vi "CreateVIPictures.vi"(8 "error in (no error)":errorcluster, 9 "Capture Target":T3=enum."Front Panel", 10 "VI 1 Screenshots":T1, 11 "Picture Save Location":path) -> (0 "error out":errorcluster, 2 "Screenshot Files":path[](array[path]))   [LabVIEW 2015, in "VIDiffScreenshots.lvlib"]
doc: "Captures .png imgaes of the VI given the path and the picture configuration."
uses:
  VIDiffScreenshots.lvlib
  Screenshot Type.ctl
  VIScreenshots.ctl
  ScreenshotInfo.ctl
  Utilities/FilePaths.ctl
  Utilities/VIDiffUtilities.lvlib
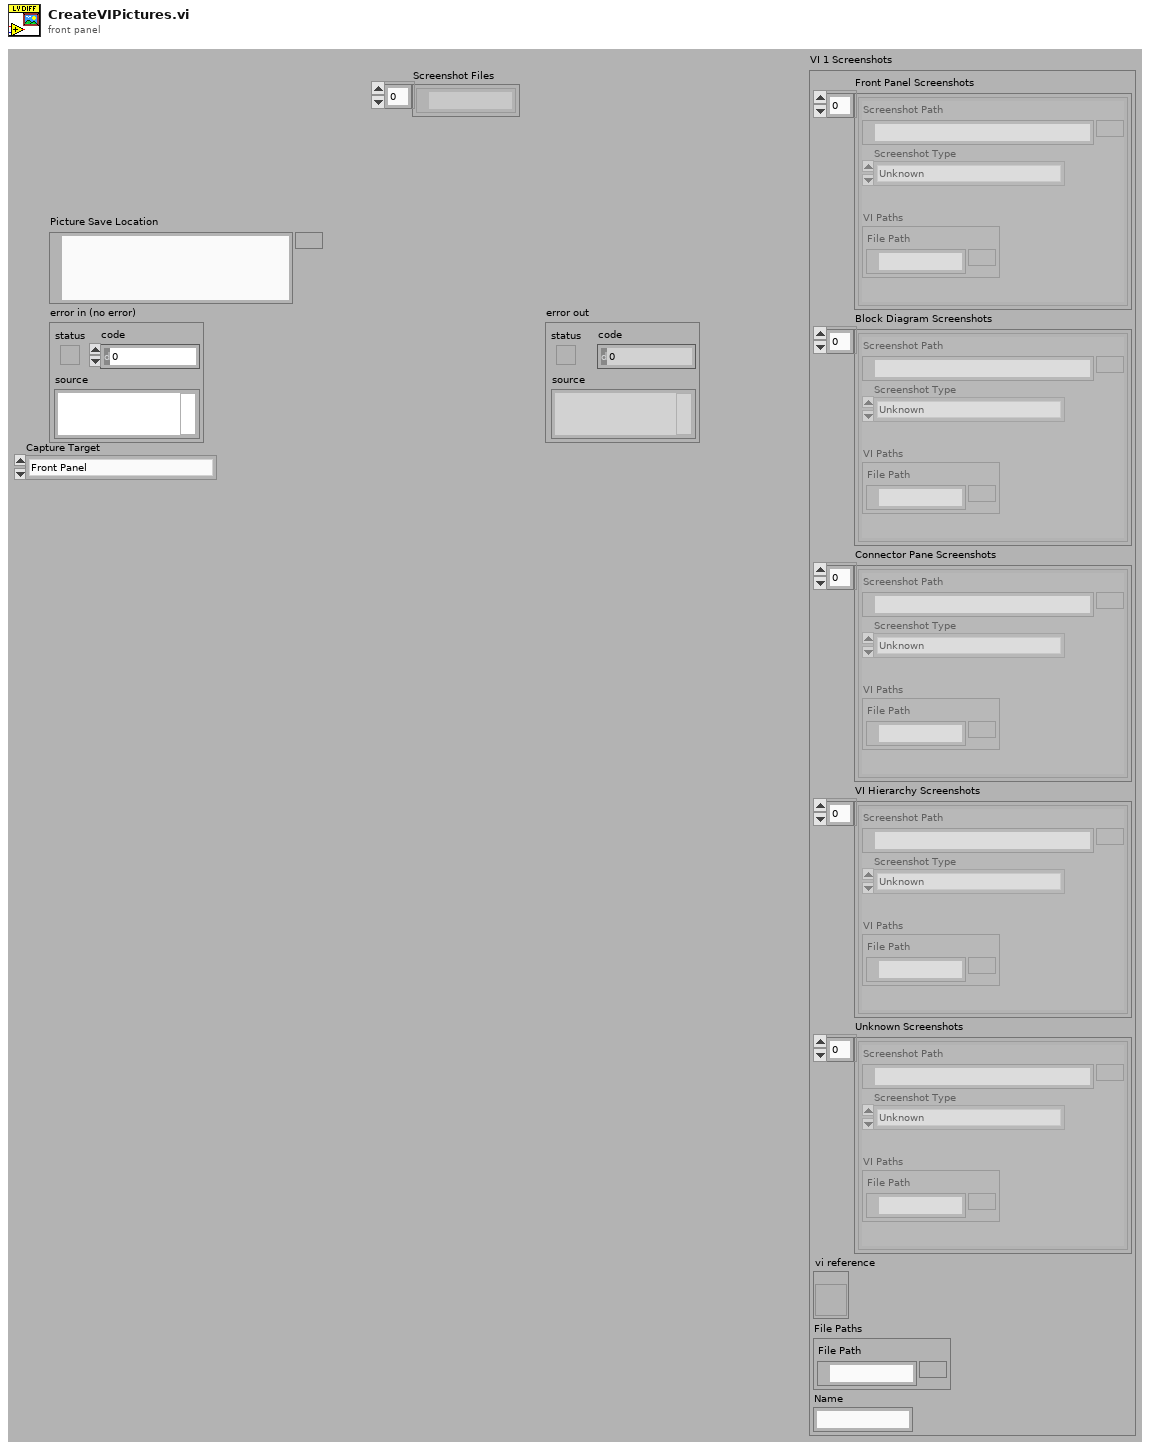
[diagram p1: front panel]
types:
  T1 = typedef "VIDiffScreenshots.lvlib/VIScreenshots.ctl" = cluster{"Front Panel Screenshots":T2[], "Block Diagram Screenshots":T2[], "Connector Pane Screenshots":T2[], "VI Hierarchy Screenshots":T2[], "Unknown Screenshots":T2[], "vi reference":refnum<vi>, "File Paths":cluster{"File Path":path}, "Name":string}
  T2 = typedef "VIDiffScreenshots.lvlib/ScreenshotInfo.ctl" = cluster{"Screenshot Path":path, "Screenshot Type":T3, "VI Paths":T4}
  T3 = typedef "VIDiffScreenshots.lvlib/Screenshot Type.ctl" = enum16{"Unknown", "Front Panel", "Connector Pane", "Block Diagram", "VI Hierarchy"}
  T4 = typedef "VIDiffUtilities.lvlib/FilePaths.ctl" = cluster{"File Path":path}
  T5 = cluster{"Printing:Custom All Controls?":bool, "Printing:Custom Connector?":bool, "Printing:Custom Control Descriptions?":bool, "Printing:Custom Control Types?":bool, "Printing:Custom Controls?":bool, "Printing:Custom Description?":bool, "Printing:Custom Diagram Hidden?":bool, "Printing:Custom Diagram Repeat?":bool, "Printing:Custom Diagram?":bool, "Printing:Custom Hierarchy?":bool, "Printing:Custom History?":bool, "Printing:Custom Panel Border?":bool, "Printing:Custom Panel?":bool, "Printing:Custom SubVIs?":bool}
  T6 = enum32{"Custom", "Standard", "Using Panel", "Using SubVI", "Complete"}
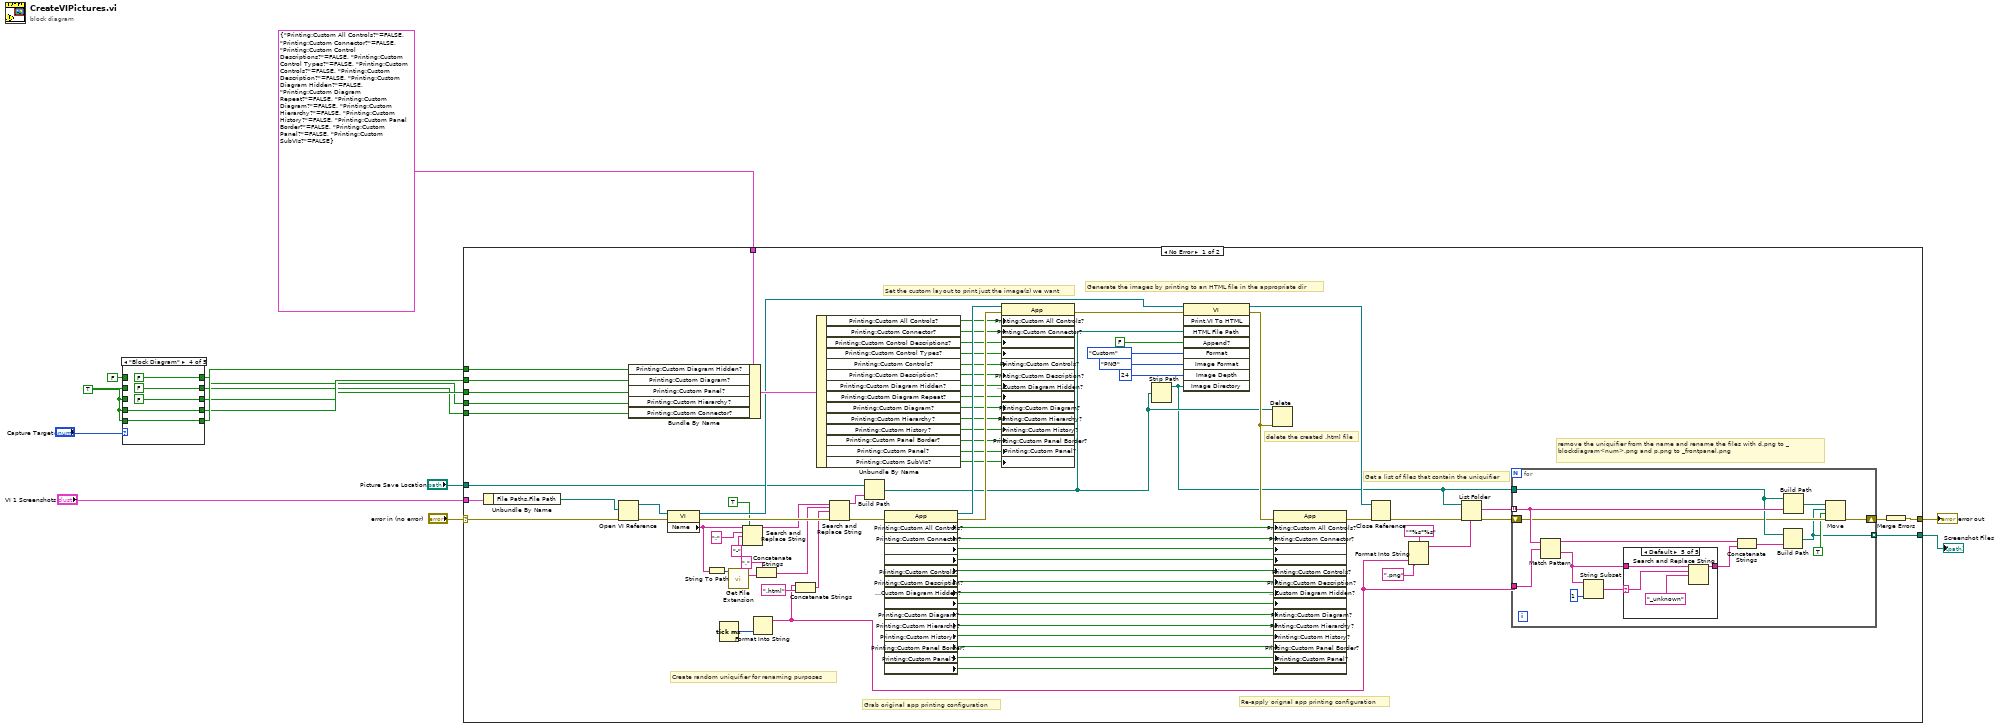
[diagram p0: block diagram]
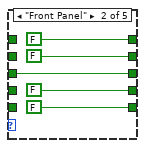
[diagram p3: hidden frame]
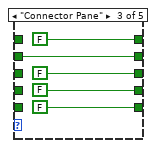
[diagram p4: hidden frame]
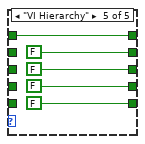
[diagram p5: hidden frame]
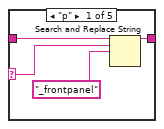
[diagram p6: hidden frame]
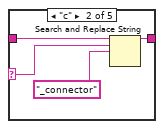
[diagram p7: hidden frame]
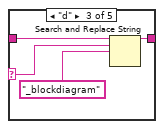
[diagram p8: hidden frame]
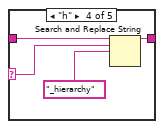
[diagram p9: hidden frame]
diagram:
  w6 = TRUE ("Capture Hierarchy?")
  n1 = case shown="\"Block Diagram\"" "Capture Target" {
    tunnel: FALSE ("Capture Hierarchy?") -> [w19 _ _ _ w35]
    tunnel: w6 -> [w18 _ w28 _ _]
    tunnel: w6 -> [w17 w24 _ _ _]
    tunnel: w6 -> [w16 _ _ w31 _]
    tunnel: w6 -> [w15 _ _ w30 _]
    tunnel: [w19 FALSE ("Capture Hierarchy?") FALSE ("Capture Hierarchy?") FALSE ("Capture Hierarchy?") w35] -> w2
    tunnel: [w18 FALSE ("Capture Connector?") w28 FALSE ("Capture Block Diagram?") FALSE ("Capture Block Diagram?")] -> w1
    tunnel: [w17 w24 FALSE ("Capture Block Diagram?") FALSE ("Capture Block Diagram?") FALSE ("Capture Block Diagram?")] -> w3
    tunnel: [w16 FALSE ("Capture Block Diagram?") FALSE ("Capture Block Diagram?") w31 FALSE ("Capture Block Diagram?")] -> w4
    tunnel: [w15 FALSE ("Capture Hidden Cases?") FALSE ("Capture Hidden Cases?") w30 FALSE ("Capture Block Diagram?")] -> w5
    frame "Unknown", Default {
    }
    frame "Front Panel" {
    }
    frame "Connector Pane" {
    }
    frame "Block Diagram" {
    }
    frame "VI Hierarchy" {
    }
  }
  n2 = case shown="No Error" "error in (no error)" {
    selector: "error in (no error)" -> [w43 w153]
    tunnel: T5 {"Printing:Custom All Controls?"=FALSE, "Printing:Custom Connector?"=FALSE, "Printing:Custom Control Descriptions?"=FALSE, "Printing:Custom Control Types?"=FALSE, "Printing:Custom Controls?"=FALSE, "Printing:Custom Description?"=FALSE, "Printing:Custom Diagram Hidden?"=FALSE, "Printing:Custom Diagram Repeat?"=FALSE, "Printing:Custom Diagram?"=FALSE, "Printing:Custom Hierarchy?"=FALSE, "Printing:Custom History?"=FALSE, "Printing:Custom Panel Border?"=FALSE, "Printing:Custom Panel?"=FALSE, "Printing:Custom SubVIs?"=FALSE} ("Content Options") -> [w118 _]
    tunnel: w5 -> [w117 _]
    tunnel: w4 -> [w116 _]
    tunnel: w3 -> [w115 _]
    tunnel: "Picture Save Location" -> [w74 _]
    tunnel: [w60 w153] -> w12
    tunnel: w2 -> [w59 _]
    tunnel: w1 -> [w58 _]
    tunnel: "VI 1 Screenshots" -> [w45 _]
    tunnel: [w41 _] -> w10
    frame No Error {
      # "remove the uniquifier from the name and rename the files with d.png to _blockdiagram<num>.png and p.png to _frontpanel.png"
      # "Get a list of files that contain the uniquifier"
      # "delete the created .html file"
      # "Create random uniquifier for renaming purposes"
      # "Re-apply orignal app printing configuration"
      # "Grab original app printing configuration"
      # "Generate the images by printing to an HTML file in the appropriate dir"
      # "Set the custom layout to print just the image(s) we want"
      n3 = Unbundle By Name(w45) -> ("File Paths.File Path"=w44:path)
      n4 = Open VI Reference(vi path=w44, error in (no error)=w43) -> (vi reference=w77:refnum<vi>, error out=w75:errorcluster)  [unwired: 4 in]
      n5 = Bundle By Name(cluster=w118, "Printing:Custom Diagram Hidden?"=w117, "Printing:Custom Diagram?"=w116, "Printing:Custom Panel?"=w115, "Printing:Custom Hierarchy?"=w59, "Printing:Custom Connector?"=w58) -> (w81:T5)
      n6 = property class="VI"(reference=w77, error in=w75) -> (reference out=w76:refnum<vi>, error out=w69:errorcluster, "Name"=w53:string)
      n7 = String To Path(string=w53) -> (path=w57:path)
      n8 = Tick Count (ms)() -> (millisecond timer value=w42:u32)
      n9 = call <vilib>:"Get File Extension.vi"("file"=w57) -> ("lowercase file extension"=w56:string)  [unwired: 6 in, 4 out]
      n10 = Search and Replace String(replace all?=TRUE ("replace all? (F)"), input string=w53, search string=":", replace string="-" ("replace string (\"\")")) -> (result string=w52:string)  [unwired: 4 in, 3 out]
      n11 = Format Into String(w42) -> (resulting string=w49:string)  [unwired: 3 in, 1 out]
      n12 = Concatenate Strings("." ("string"), w56) -> (w54:string)
      n13 = Concatenate Strings(w49, ".html" ("regular expression")) -> (w48:string)
      n14 = Unbundle By Name(w81) -> ("Printing:Custom All Controls?"=w95:bool, "Printing:Custom Connector?"=w94:bool, "Printing:Custom Control Descriptions?"=w93:bool, "Printing:Custom Control Types?"=w92:bool, "Printing:Custom Controls?"=w91:bool, "Printing:Custom Description?"=w90:bool, "Printing:Custom Diagram Hidden?"=w89:bool, "Printing:Custom Diagram Repeat?"=w88:bool, "Printing:Custom Diagram?"=w87:bool, "Printing:Custom Hierarchy?"=w86:bool, "Printing:Custom History?"=w85:bool, "Printing:Custom Panel Border?"=w84:bool, "Printing:Custom Panel?"=w83:bool, "Printing:Custom SubVIs?"=w82:bool)
      n15 = Search and Replace String(input string=w52, search string=w54, replace string=w48, error in=w69) -> (result string=w70:string, error out=w68:errorcluster)  [unwired: 4 in, 2 out]
      n16 = Build Path(base path=w74, name or relative path=w70) -> (appended path=w71:path)
      n17 = property class="App"(error in=w68) -> (reference out=w100:refnum<vi>, error out=w99:errorcluster, "Printing:Custom All Controls?"=w101:bool, "Printing:Custom Connector?"=w102:bool, "Printing:Custom Control Descriptions?"=w103:bool, "Printing:Custom Control Types?"=w104:bool, "Printing:Custom Controls?"=w105:bool, "Printing:Custom Description?"=w106:bool, "Printing:Custom Diagram Hidden?"=w107:bool, "Printing:Custom Diagram Repeat?"=w108:bool, "Printing:Custom Diagram?"=w109:bool, "Printing:Custom Hierarchy?"=w110:bool, "Printing:Custom History?"=w111:bool, "Printing:Custom Panel Border?"=w112:bool, "Printing:Custom Panel?"=w113:bool, "Printing:Custom List of SubVIs?"=w114:bool)  [unwired: 1 in]
      n18 = property class="App"(reference=w100, error in=w99, "Printing:Custom All Controls?"=w95, "Printing:Custom Connector?"=w94, "Printing:Custom Control Descriptions?"=w93, "Printing:Custom Control Types?"=w92, "Printing:Custom Controls?"=w91, "Printing:Custom Description?"=w90, "Printing:Custom Diagram Hidden?"=w89, "Printing:Custom Diagram Repeat?"=w88, "Printing:Custom Diagram?"=w87, "Printing:Custom Hierarchy?"=w86, "Printing:Custom History?"=w85, "Printing:Custom Panel Border?"=w84, "Printing:Custom Panel?"=w83, "Printing:Custom List of SubVIs?"=w82) -> (error out=w98:errorcluster)  [unwired: 1 out]
      n19 = Strip Path(path=w71) -> (stripped path=w63:path)  [unwired: 1 out]
      n20 = invoke class="VI" method="Print.VI To HTML"(reference=w76, error in=w98, "HTML File Path"=w71, "Append?"=FALSE, "Format"=T6."Custom", "Image Format"=enum32{"PNG", "JPEG", "GIF"}."PNG" ("Image Format (jpeg)"), "Image Depth"=24, "Image Directory"=w63) -> (reference out=w72:refnum<vi>, error out=w78:errorcluster)  [unwired: 1 in, 7 out]
      n21 = Delete(path (use dialog)=w71, error in=w78) -> ()  [unwired: 3 in, 3 out]
      n22 = property class="App"(error in=w78, "Printing:Custom All Controls?"=w101, "Printing:Custom Connector?"=w102, "Printing:Custom Control Descriptions?"=w103, "Printing:Custom Control Types?"=w104, "Printing:Custom Controls?"=w105, "Printing:Custom Description?"=w106, "Printing:Custom Diagram Hidden?"=w107, "Printing:Custom Diagram Repeat?"=w108, "Printing:Custom Diagram?"=w109, "Printing:Custom Hierarchy?"=w110, "Printing:Custom History?"=w111, "Printing:Custom Panel Border?"=w112, "Printing:Custom Panel?"=w113, "Printing:Custom List of SubVIs?"=w114) -> (error out=w73:errorcluster)  [unwired: 1 in, 1 out]
      n23 = Close Reference(reference=w72, error in (no error)=w73) -> (error out=w66:errorcluster)
      n24 = Format Into String(format string="*%s*%s" ("Format String"), w49, ".png" ("input 2")) -> (resulting string=w65:string)  [unwired: 2 in, 1 out]
      n25 = List Folder(path=w63, pattern=w65, error in=w66) -> (filenames=w62:string[], error out=w61:errorcluster)  [unwired: 1 in, 2 out]
      n26 = for {
        tunnel: w63 -> [w125]
        tunnel: w62 -> [w126] mode=indexing
        tunnel: w49 -> [w123]
        shift-right: [w121] -> w51
        shift-left: w61 -> [w122]
        tunnel: [w119] -> w41 mode=indexing
        n27 = Match Pattern(string=w126, regular expression=w123) -> (before substring=w128:string, after substring=w130:string)  [unwired: 1 in, 2 out]
        n28 = String Subset(string=w130, length (rest)=1 ("length (rest)")) -> (substring=w131:string)  [unwired: 1 in]
        n29 = case shown="Default" w131 {
          selector: w131 -> [w135 w139 w143 w147 w151]
          tunnel: w130 -> [w136 w140 w144 w148 w152]
          tunnel: [w133 w137 w141 w145 w149] -> w129
          frame "p" {
            n30 = Search and Replace String(input string=w136, search string=w135, replace string="_frontpanel" ("replace string (\"\")")) -> (result string=w133:string)  [unwired: 5 in, 3 out]
          }
          frame "c" {
            n31 = Search and Replace String(input string=w140, search string=w139, replace string="_connector" ("replace string (\"\")")) -> (result string=w137:string)  [unwired: 5 in, 3 out]
          }
          frame "d" {
            n32 = Search and Replace String(input string=w144, search string=w143, replace string="_blockdiagram" ("replace string (\"\")")) -> (result string=w141:string)  [unwired: 5 in, 3 out]
          }
          frame "h" {
            n33 = Search and Replace String(input string=w148, search string=w147, replace string="_hierarchy" ("replace string (\"\")")) -> (result string=w145:string)  [unwired: 5 in, 3 out]
          }
          frame Default {
            n34 = Search and Replace String(input string=w152, search string=w151, replace string="_unknown" ("replace string (\"\")")) -> (result string=w149:string)  [unwired: 5 in, 3 out]
          }
        }
        n35 = Concatenate Strings(w128, w129) -> (w127:string)
        n36 = Build Path(base path=w125, name or relative path=w127) -> (appended path=w119:path)
        n37 = Build Path(base path=w125, name or relative path=w126) -> (appended path=w124:path)
        n38 = Move(source path=w124, error in=w122, 9:TRUE ("overwrite (F)"), 10:w119) -> (error out=w121:errorcluster)  [unwired: 1 in, 2 out]
      }
      n39 = Merge Errors(w51) -> (w60:errorcluster)
    }
    frame Error {
    }
  }
  "error out" <- w12
  "Screenshot Files" <- w10
